vi "only flame and temp.vi"() -> ()   [LabVIEW 2017]
panel:
  out "Low Lighing":bool
  out "High Temperature":bool
  out "Low Temperature":bool
  out "Thermometer":dbl(slide) scale=0.0..100.0
  out "LDR Output (V)":dbl
  out "Temperatue (C)":dbl
  out "Temperature in (mV)":dbl
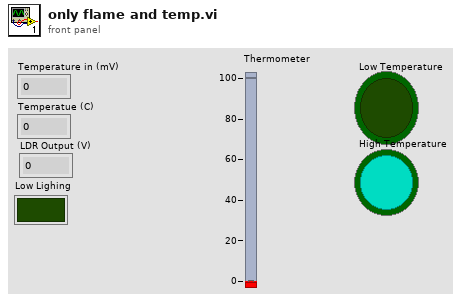
[diagram p1: front panel]
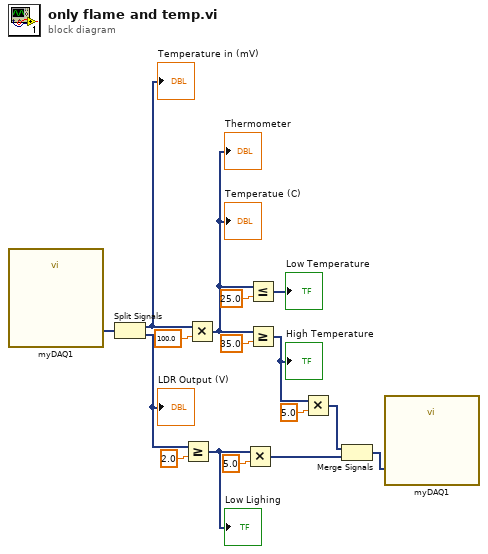
[diagram p0: block diagram]
diagram:
  n1 = call "myDAQ1"() -> ("data"=w4:dynamicdata)  [unwired: 16 in, 3 out]
  n2 = Split Signals(w4) -> (w16:dynamicdata, w14:dynamicdata)  [unwired: 2 in]
  "Temperature in (mV)" <- w16
  "LDR Output (V)" <- w14
  n3 = Greater Or Equal?(x=w14, y=2.0) -> (x >= y?=w6:dynamicdata)
  "Low Lighing" <- w6
  n4 = Multiply(x=w16, y=100.0) -> (x*y=w9:dynamicdata)
  "Temperatue (C)" <- w9
  "Thermometer" <- w9
  n5 = Multiply(x=w6, y=5.0) -> (x*y=w2:dynamicdata)
  n6 = Less Or Equal?(x=w9, y=25.0) -> (x <= y?=→"Low Temperature":dynamicdata)
  n7 = Greater Or Equal?(x=w9, y=35.0) -> (x >= y?=w8:dynamicdata)
  "High Temperature" <- w8
  n8 = Multiply(x=w8, y=5.0) -> (x*y=w1:dynamicdata)
  n9 = Merge Signals(w1, w2) -> (w3:dynamicdata)
  n10 = call "myDAQ1"("data"=w3) -> ()  [unwired: 16 in, 3 out]
